vi "Write.vi"(8 "error in (no error)":errorcluster, 9 "Options":T2, 10 "Anything":variant, 11 "Tree in":refnum<vi>) -> (0 "error out":errorcluster, 2 "Tree Items":T1[](array[typedef]), 3 "Tree out":refnum<vi>)   [LabVIEW 2020, in "BlueVariantView.lvlib"]
doc: "This method will overwrite all data in your tree control.\n\nOptions.Colorize --> If yes, this will colorize the tree text to match data type"
uses:
  BlueVariantView.lvlib
  Typedefs/Options.ctl
  Typedefs/TreeData.ctl
  Support/LoopData.ctl
  Defer Panel Updates/SubVIs/defer panel updates Controlref step1.vi
  Defer Panel Updates/SubVIs/defer panel updates step2.vi
  Defer Panel Updates/Defer Panel Updates BVV.lvlib
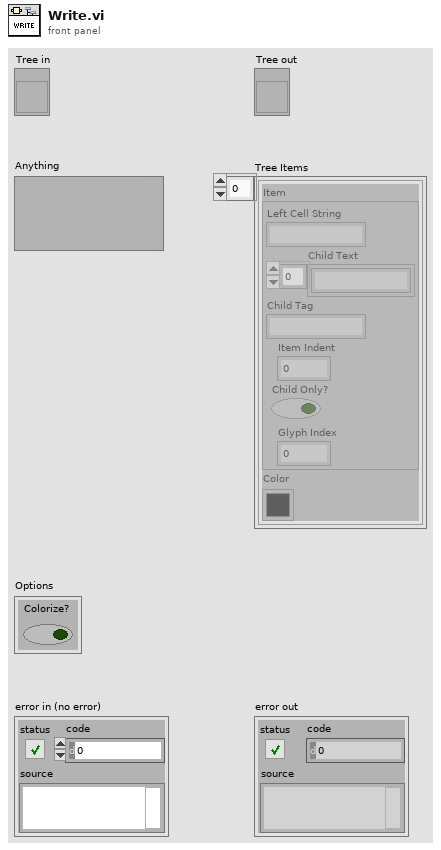
[diagram p1: front panel]
types:
  T1 = typedef "BlueVariantView.lvlib/TreeData.ctl" = cluster{"Item":cluster{"Left Cell String":string, "Child Text":string[], "Child Tag":string, "Item Indent":i32, "Child Only?":bool, "Glyph Index":i32}, "Color":u32}
  T2 = typedef "BlueVariantView.lvlib/Options.ctl" = cluster{"Colorize?":bool}
  T3 = typedef "BlueVariantView.lvlib/LoopData.ctl" = cluster{"Tags":set{string}}
  T4 = typedef "Defer Panel Updates BVV.lvlib/defer panel updates data.ctl" = cluster{"Owning VI":refnum<vi>, "Front Panel":refnum<vi>, "performed?":bool}
  T5 = cluster{"Left Cell String":string, "Child Text":string[], "Child Tag":string, "Item Indent":i32, "Child Only?":bool, "Glyph Index":i32}
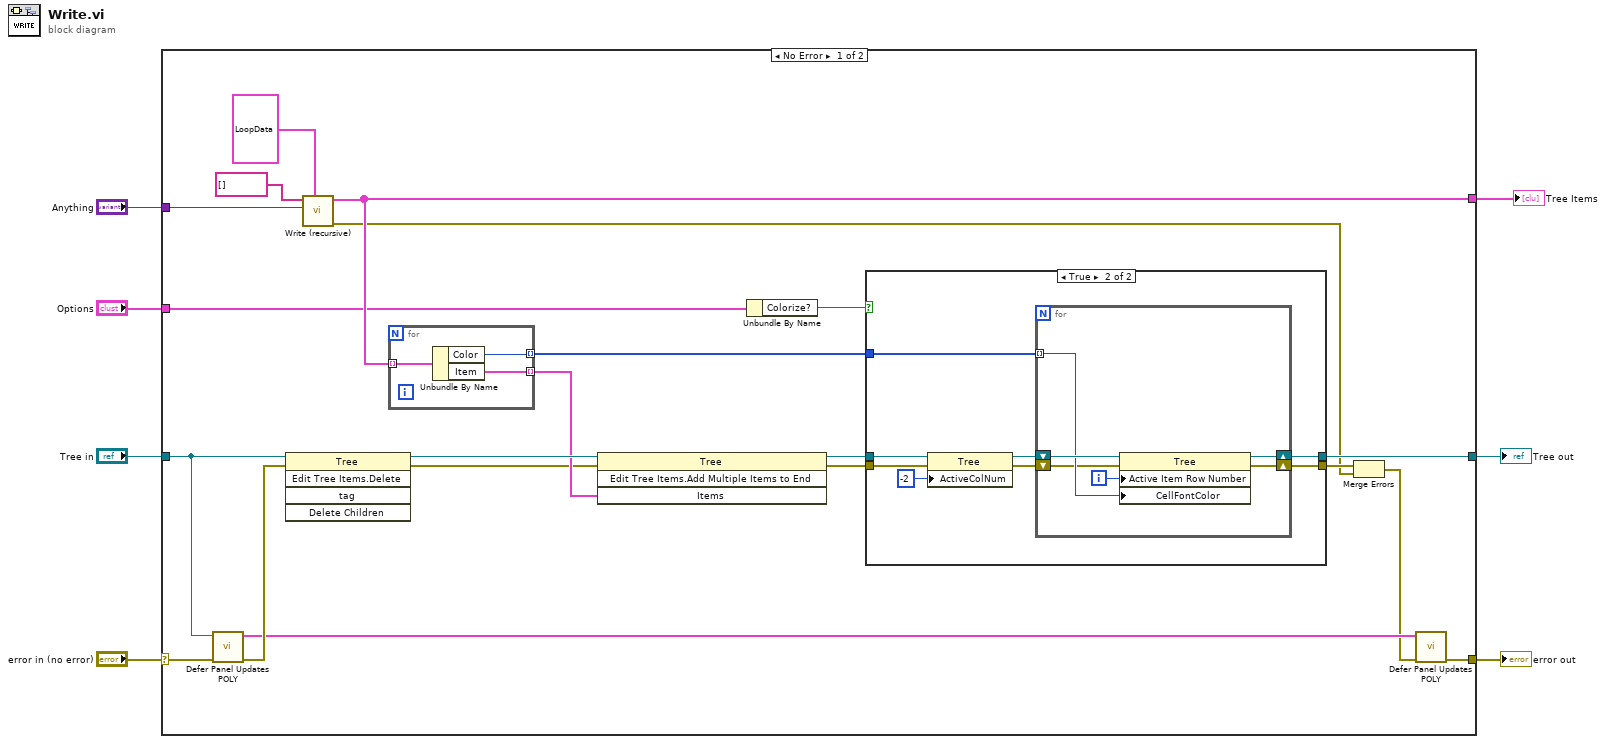
[diagram p0: block diagram]
diagram:
  n1 = case shown="No Error" "error in (no error)" {
    selector: "error in (no error)" -> [w26 w49]
    tunnel: "Anything" -> [w28 _]
    tunnel: "Tree in" -> [w27 w48]
    tunnel: [w11 w49] -> w4
    tunnel: [w21 _] -> w3
    tunnel: [w16 w48] -> w2
    tunnel: "Options" -> [w13 _]
    frame No Error {
      n2 = call-poly "Defer Panel Updates POLY.vi"("error in (no error)"=w26, "control reference"=w27) -> ("error out"=w25:errorcluster, "Refs"=w24:T4)  [unwired: 8 in]
      n3 = invoke class="Tree" method="Edit Tree Items.Delete"(reference=w27, error in=w25) -> (reference out=w20:refnum<vi>, error out=w15:errorcluster)  [unwired: 3 in, 3 out]
      n4 = call "Write (recursive).vi"("LoopData in"=T3 {"Tags"={}}, "Anything"=w28, "TagPath"=string[] []) -> ("error out"=w9:errorcluster, "Tree Items"=w21:T1[])  [unwired: 6 in, 1 out]
      n5 = for {
        tunnel: w21 -> [w31] mode=indexing
        tunnel: [w30] -> w17 mode=indexing
        tunnel: [w29] -> w19 mode=indexing
        n6 = Unbundle By Name(w31) -> ("Color"=w30:u32, "Item"=w29:T5)
      }
      n7 = invoke class="Tree" method="Edit Tree Items.Add Multiple Items to End"(reference=w20, error in=w15, "Items"=w19) -> (reference out=w18:refnum<vi>, error out=w14:errorcluster)  [unwired: 1 in, 2 out]
      n8 = Unbundle By Name(w13) -> ("Colorize?"=w12:bool)
      n9 = case shown="True" w12 {
        tunnel: w18 -> [w33 w39]
        tunnel: w17 -> [_ w38]
        tunnel: [w33 w37] -> w16
        tunnel: w14 -> [w32 w36]
        tunnel: [w32 w34] -> w10
        frame False {
        }
        frame True {
          n10 = property class="Tree"(reference=w39, error in=w36, "ActiveColNum"=-2 ("Active Cell:Active Column Number")) -> (reference out=w40:refnum<vi>, error out=w35:errorcluster)
          n11 = for {
            shift-right: [w45] -> w37
            shift-left: w40 -> [w47]
            tunnel: w38 -> [w44] mode=indexing
            shift-right: [w42] -> w34
            shift-left: w35 -> [w43]
            i -> [w46]
            n12 = property class="Tree"(reference=w47, error in=w43, "Active Item Row Number"=w46, "CellFontColor"=w44) -> (reference out=w45:refnum<vi>, error out=w42:errorcluster)
          }
        }
      }
      n13 = Merge Errors(w10, w9) -> (w8:errorcluster)
      n14 = call-poly "Defer Panel Updates POLY.vi"("error in (no error)"=w8, "Refs"=w24) -> ("error out"=w11:errorcluster)  [unwired: 9 in]
    }
    frame Error {
    }
  }
  "error out" <- w4
  "Tree out" <- w2
  "Tree Items" <- w3
